vi "NotifyIcon - Example.vi"() -> ()   [LabVIEW 2018]
uses:
  TypeDefs/NotifyIcon Events.ctl
  TypeDefs/NotifyIcon Event Registration Actions.ctl
panel:
  in  "Text":string="Baloon Tip Text"
  in  "Title":string="Balloon Tip"
  in  "Icon (None)":i32(ring)=1 items=["None", "Info", "Warning", "Error"]
  in  "Show Balloon Tip":bool
  in  "stop":bool
  in  "Icon File Path":path=path "C:/Program Files/National Instruments/LabVIEW 2009/applibs/lvapp.ico"
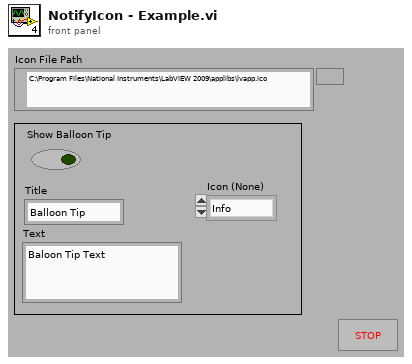
[diagram p1: front panel]
types:
  T1 = typedef "NotifyIcon Event Registration Actions.ctl" = enum16{"Initial Event Registration", "Add to Event Registration", "Destroy Events and Re-register"}
  T2 = typedef "NotifyIcon Events.ctl" = enum16{"BalloonTipClicked", "BalloonTipClosed", "BalloonTipShown", "Click", "Disposed", "DoubleClick", "MouseClick", "MouseDoubleClick", "MouseDown", "MouseMove", "MouseUp", "MenuItemClick", "MenuItemSelect"}
  T3 = typedef "NotifyIcon Event Data.ctl" = cluster{"NotifyIcon Event":T2, "Data String":string}
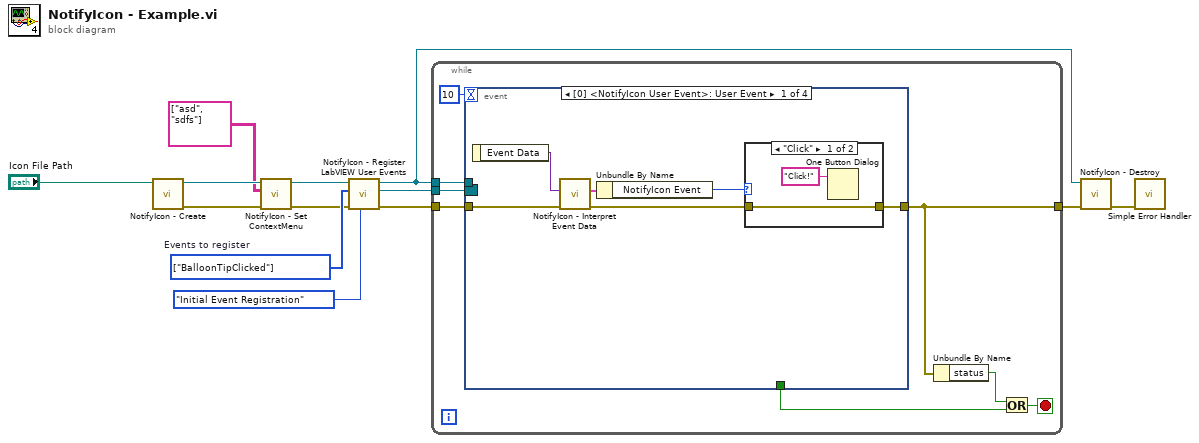
[diagram p0: block diagram]
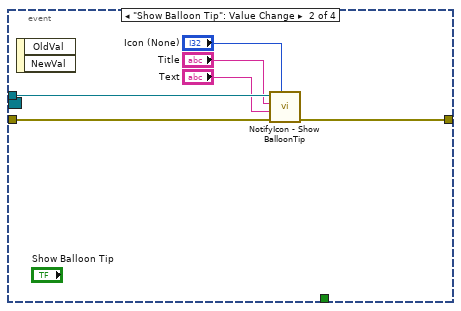
[diagram p3: hidden frame]
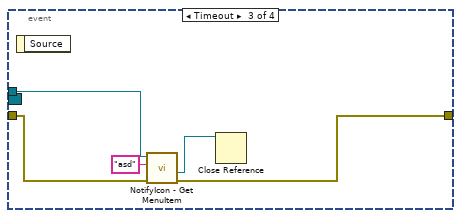
[diagram p4: hidden frame]
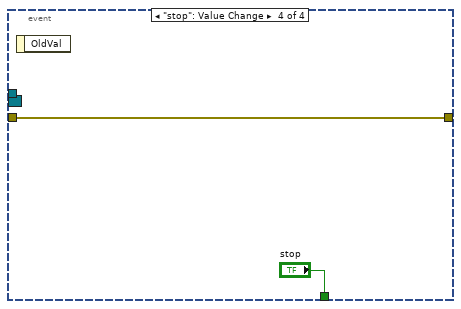
[diagram p5: hidden frame]
diagram:
  w12 = T2[] [enum."BalloonTipClicked"] items=["BalloonTipClicked", "BalloonTipClosed", "BalloonTipShown", "Click", "Disposed", "DoubleClick", "MouseClick", "MouseDoubleClick", "MouseDown", "MouseMove", "MouseUp", "MenuItemClick", "MenuItemSelect"]  # Events to register
  n1 = call "NotifyIcon - Create.vi"("Icon File Path"="Icon File Path") -> ("error out"=w5:errorcluster, "NotifyIcon reference"=w3:refnum<k24>)  [unwired: 9 in]
  n2 = call "NotifyIcon - Set ContextMenu.vi"("error in"=w5, "Context Menu"=string[][] [["asd"], ["sdfs"]], "NotifyIcon reference in"=w3) -> ("error out"=w4:errorcluster, "NotifyIcon reference out"=w2:refnum<k24>)  [unwired: 7 in]
  n3 = call "NotifyIcon - Register LabVIEW User Events.vi"("Action"=NotifyIcon_Event_Registration_Actions."Initial Event Registration", "error in"=w4, "Events to register"=w12, "NotifyIcon reference in"=w2) -> ("error out"=w9:errorcluster, "Event Registration Refnum"=w10:refnum<event-registration>, "NotifyIcon reference out"=w6:refnum<k24>)  [unwired: 5 in]
  n4 = while {
    tunnel: w10 -> [w21]
    tunnel: w6 -> [w20]
    tunnel: w9 -> [w19]
    tunnel: [w15] -> w8
    stop <- w16 stop-if-true
    n5 = event shown="[0] <NotifyIcon User Event>: User Event" {
      selector: w21 -> [_ _ _ _]
      dyn-events: _ -> [_ _ _ _]
      timeout: 10 -> [_ _ _ _]
      tunnel: w20 -> [_ w35 w40 _]
      tunnel: w19 -> [w27 w36 w41 w42]
      tunnel: [_ _ _ "stop"] -> w18
      tunnel: [w22 w31 w39 w42] -> w15
      event User Event {
        n6 = event-data() -> ("Event Data"=w26:variant)  [unwired: 1 in]
        n7 = call "NotifyIcon - Interpret Event Data.vi"("error in"=w27, "NotifyIcon Event Data"=w26) -> ("error out"=w23:errorcluster, "NotifyIcon Event Data"=w25:T3)  [unwired: 8 in]
        n8 = Unbundle By Name(w25) -> ("NotifyIcon Event"=w24:T2)
        n9 = case shown="\"Click\"" w24 {
          tunnel: w23 -> [w28 w30]
          tunnel: [w28 w30] -> w22
          frame "Click" {
            n10 = One Button Dialog(message="Click!") -> ()  [unwired: 1 in, 1 out]
          }
          frame Default {
          }
        }
      }
      event "Show Balloon Tip": Value Change {
        n11 = event-data() -> ()  [unwired: 1 in, 2 out]
        n12 = call "NotifyIcon - Show BalloonTip.vi"("Icon (None)"="Icon (None)", "error in"=w36, "Text"="Text", "Title"="Title", "NotifyIcon reference in"=w35) -> ("error out"=w31:errorcluster)  [unwired: 5 in, 1 out]
      }
      event Timeout {
        n13 = event-data() -> ()  [unwired: 1 in, 1 out]
        n14 = call "NotifyIcon - Get MenuItem.vi"("error in"=w41, "Context MenuItem"="asd", "NotifyIcon reference in"=w40) -> ("error out"=w39:errorcluster, "MenuItem reference"=w38:refnum<k24>)  [unwired: 6 in, 1 out]
        n15 = Close Reference(reference=w38) -> ()  [unwired: 1 in, 1 out]
      }
      event "stop": Value Change {
        n16 = event-data() -> ()  [unwired: 1 in, 1 out]
      }
    }
    n17 = Unbundle By Name(w15) -> ("status"=w17:bool)
    n18 = Or(x=w17, y=w18) -> (x .or. y?=w16:bool)
  }
  n19 = call "NotifyIcon - Destroy.vi"("error in"=w8, "NotifyIcon reference"=w6) -> ("error out"=w7:errorcluster)  [unwired: 9 in]
  n20 = call <vilib>:"Simple Error Handler.vi"("error in (no error)"=w7) -> ()  [unwired: 4 in, 5 out]
